vi "Ficheros.vi"() -> ()   [LabVIEW 2020]
uses:
  <vilib>/ErrorRing/Error Ring.xnode
panel:
  in  "Combo Box":string(combo)
  in  "Tipo de Archivo":string(combo)
  in  "Nombre Archivo":string
  in  "Direccion":path
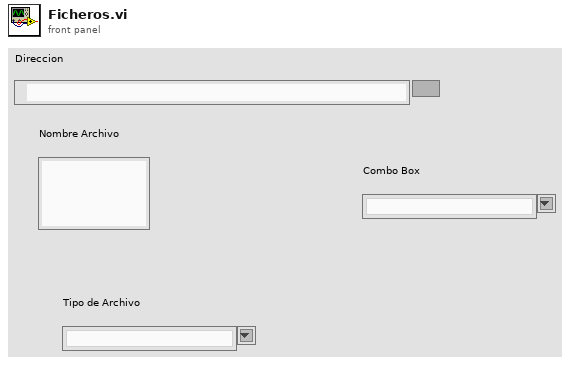
[diagram p1: front panel]
types:
  T1 = enum16{"open", "replace", "create", "open or create", "replace or create", "replace or create with confirmation"}
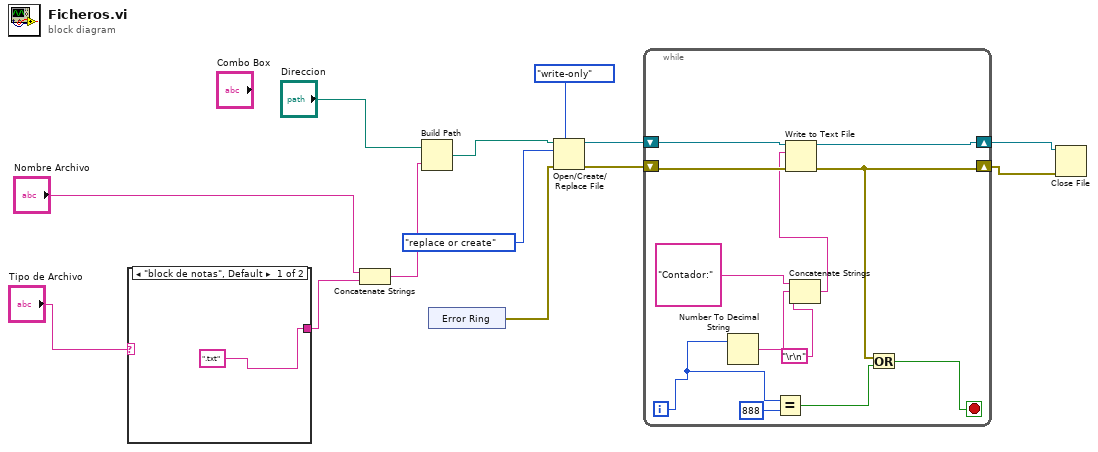
[diagram p0: block diagram]
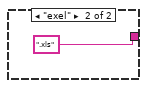
[diagram p2: hidden frame]
diagram:
  n1 = case shown="\"block de notas\", Default" "Tipo de Archivo" {
    tunnel: [".txt" ".xls"] -> w10
    frame "block de notas", Default {
    }
    frame "exel" {
    }
  }
  n2 = Concatenate Strings("Nombre Archivo", w10) -> (w9:string)
  n3 = Build Path(base path="Direccion", name or relative path=w9) -> (appended path=w8:path)
  n4 = xnode "Error Ring"() -> ("error out"=w5:errorcluster)
  n5 = Open/Create/Replace File(file path (use dialog)=w8, error in=w5, operation (0:open)=T1."replace or create", access (0:read/write)=enum16{"read/write", "read-only", "write-only"}."write-only") -> (refnum out=w4:refnum<file>, error out=w3:errorcluster)  [unwired: 2 in, 1 out]
  n6 = while {
    shift-right: [w25] -> w2
    shift-left: w4 -> [w27]
    shift-right: [w17] -> w1
    shift-left: w3 -> [w26]
    i -> [w20]
    stop <- w16 stop-if-true
    n7 = Number To Decimal String(number=w20) -> (decimal integer string=w23:string)  [unwired: 1 in]
    n8 = Equal?(x=w20, y=888) -> (x = y?=w18:bool)
    n9 = Concatenate Strings("Contador:", w23, "\r\n") -> (w21:string)
    n10 = Write to Text File(file (use dialog)=w27, text=w21, error in=w26) -> (refnum out=w25:refnum<file>, error out=w17:errorcluster)  [unwired: 1 in, 1 out]
    n11 = Or(x=w17, y=w18) -> (x .or. y?=w16:bool)
  }
  n12 = Close File(refnum=w2, error in=w1) -> ()  [unwired: 2 out]
